vi "source Write.vi"(4 "error in (no error)":errorcluster, 5 "Value":cluster{"connect":bool, "Z_Source":T1}, 6 "Container State":T4, 7 "Display State In":T2={"Z_Source"={"connect"=FALSE, "Z_Source"=enum."initialize"}, "Write"=FALSE, "Z1_ind"=0, "button state"=0, "reset_timer"=FALSE, "load_timer"=FALSE, "end_timer"=TRUE} {"button state" items=["init", "not connect", "local disabled", "local hand", "set hand", "hand", "set auto", "auto", "dist"]}) -> (0 "error out":errorcluster, 3 "Display State Out":T2={"Z_Source"={"connect"=FALSE, "Z_Source"=enum."initialize"}, "Write"=FALSE, "Z1_ind"=0, "button state"=0, "reset_timer"=FALSE, "load_timer"=FALSE, "end_timer"=TRUE} {"button state" items=["init", "not connect", "local disabled", "local hand", "set hand", "hand", "set auto", "auto", "dist"]})   [LabVIEW 2019, in "Heating.lvlib" / "Z_Hswitch_little.xctl"]
uses:
  Z_Hswitch_little.xctl
  <vilib>/_xctls/Container State.ctl
  State.ctl
  Z_source.ctl
  AutoButton_state.ctl
  <vilib>/_xctls/XControlSupport.lvlib
  Heating.lvlib
panel:
  # "Replace the Value Control below with a Control of desired type.\nDo not remove this Control or the others from the connector pane.\nDo not change the connector pane pattern.\nThe Value control should always be the third terminal from top on the input side in the connector pane."
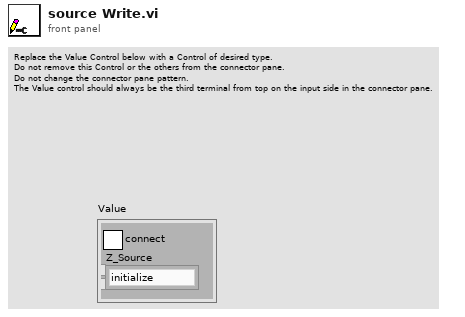
[diagram p1: front panel]
types:
  T1 = typedef "Heating.lvlib/Z_source.ctl" = enum8{"initialize", "local disabled", "local hand", "hand", "auto", "dist"}
  T2 = typedef "Heating.lvlib/Z_Hswitch_little.xctl/State.ctl" = cluster{"Z_Source":cluster{"connect":bool, "Z_Source":T1}, "Write":bool, "Z1_ind":u8, "button state":T3, "reset_timer":bool, "load_timer":bool, "end_timer":bool}
  T3 = typedef "Heating.lvlib/Z_Hswitch_little.xctl/AutoButton_state.ctl" = u16
  T4 = typedef "XControlSupport.lvlib/Container State.ctl" = cluster{"Indicator?":bool, "Run Mode?":bool, " Refnum":refnum<vi>}
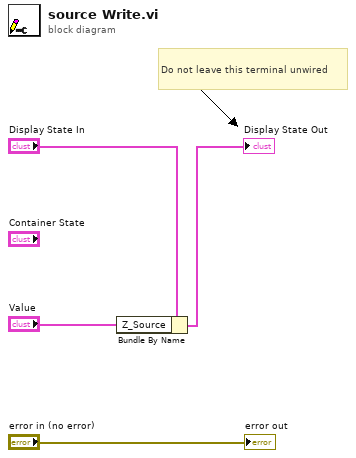
[diagram p0: block diagram]
diagram:
  # "Do not leave this terminal unwired"
  n1 = Bundle By Name(cluster="Display State In", "Z_Source"="Value") -> (→"Display State Out":T2)
  "error out" <- "error in (no error)"
